vi "Test_Read_file_to_2_1D_arrays.vi"() -> ()   [LabVIEW 2020]
uses:
  #typedef_Program_Data.ctl
  #typedef_English_Teacher_States.ctl
panel:
  out "ProgramData":T1
  in  "Path":path
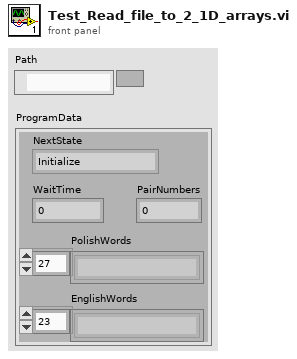
[diagram p1: front panel]
types:
  T1 = typedef "#typedef_Program_Data.ctl" = cluster{"WaitTime":dbl, "PolishWords":string[], "EnglishWords":string[], "PairNumbers":u32, "NextState":T2}
  T2 = typedef "#typedef_English_Teacher_States.ctl" = enum16{"Initialize", "Idle", "Learning_1", "Learning_2", "Learning_3", "Test_1", "Test_2", "Test_3", "Test_4", "Stop", "Exit"}
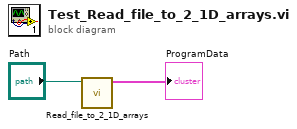
[diagram p0: block diagram]
diagram:
  n1 = call "Read_file_to_2_1D_arrays.vi"("Path"="Path") -> ("ProgramData"=→"ProgramData":T1)  [unwired: 9 in, 1 out]
